vi "Write Datalog.vi"(8 "error in":errorcluster, 9 "Model Name":T1, 10 "Results":T2, 11 "file path (dialog if empty)":path) -> (0 "error in":errorcluster)   [LabVIEW 2017]
uses:
  controls/AC Results.ctl
  controls/Model Name.ctl
  <vilib>/Utility/file.llb/Write Delimited Spreadsheet (string).vi
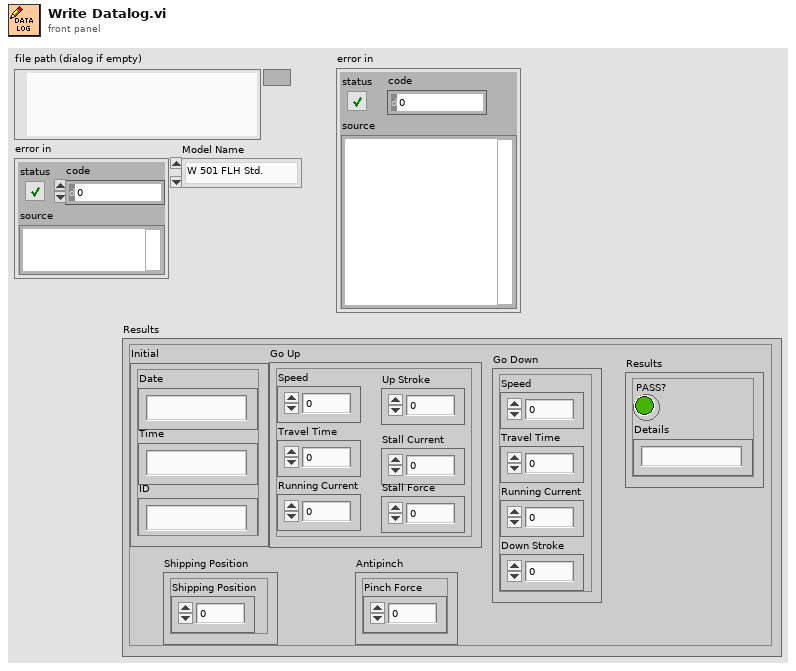
[diagram p1: front panel]
types:
  T1 = typedef "Model Name.ctl" = enum16{"W 501 FLH Std.", "W 501 FRH Std.", "W 601 FR RH Std", "W 601 FR LH Std", "W 601 RR RH Std", "W 601 RR LH Std", "W 601 FR RH AP", "W 601 FR LH AP", "W 601 RR RH AP", "W 601 RR LH AP"}
  T2 = typedef "AC Results.ctl" = cluster{"Initial":cluster{"Date":string, "Time":string, "ID":string}, "Go Up":cluster{"Speed":dbl, "Travel Time":dbl, "Running Current":dbl, "Up Stroke":dbl, "Stall Current":dbl, "Stall Force":dbl}, "Go Down":cluster{"Speed":dbl, "Travel Time":dbl, "Running Current":dbl, "Down Stroke":dbl}, "Shipping Position":cluster{"Shipping Position":dbl}, "Results":cluster{"PASS?":bool, "Details":string}, "Antipinch":cluster{"Pinch Force":dbl}}
  T3 = cluster{"Date":string, "Time":string, "ID":string, string, string, string, string, string, string, string, string, string, string, string, string, string, string, "Details":string}
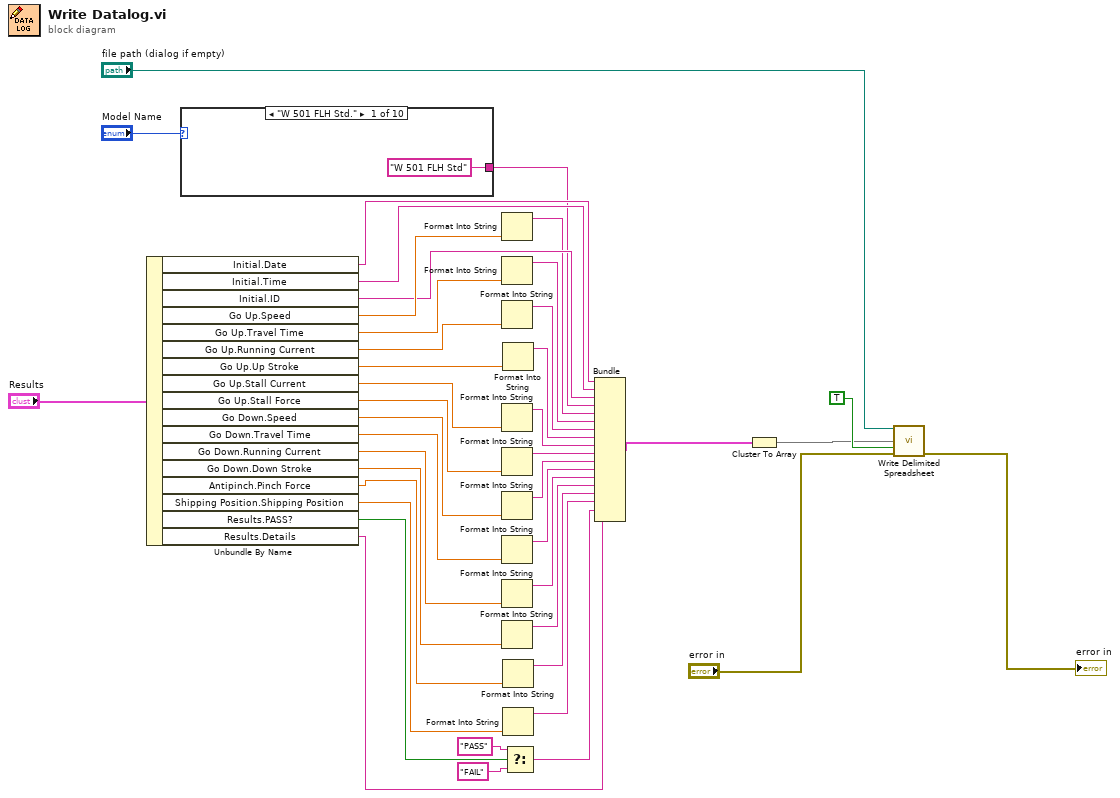
[diagram p0: block diagram]
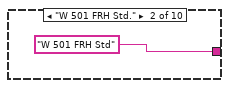
[diagram p2: hidden frame]
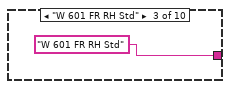
[diagram p3: hidden frame]
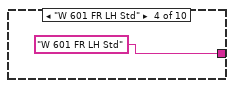
[diagram p4: hidden frame]
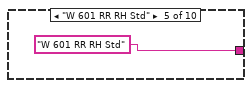
[diagram p5: hidden frame]
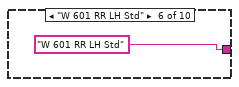
[diagram p6: hidden frame]
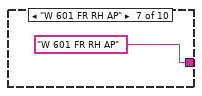
[diagram p7: hidden frame]
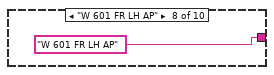
[diagram p8: hidden frame]
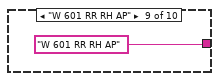
[diagram p9: hidden frame]
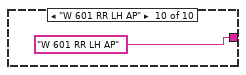
[diagram p10: hidden frame]
diagram:
  n1 = Unbundle By Name("Results") -> ("Initial.Date"=w26:string, "Initial.Time"=w25:string, "Initial.ID"=w24:string, "Go Up.Speed"=w34:dbl, "Go Up.Travel Time"=w33:dbl, "Go Up.Running Current"=w32:dbl, "Go Up.Up Stroke"=w11:dbl, "Go Up.Stall Current"=w31:dbl, "Go Up.Stall Force"=w30:dbl, "Go Down.Speed"=w29:dbl, "Go Down.Travel Time"=w28:dbl, "Go Down.Running Current"=w27:dbl, "Go Down.Down Stroke"=w9:dbl, "Antipinch.Pinch Force"=w4:dbl, "Shipping Position.Shipping Position"=w3:dbl, "Results.PASS?"=w8:bool, "Results.Details"=w7:string)
  n2 = case shown="\"W 501 FLH Std.\"" "Model Name" {
    tunnel: ["W 501 FLH Std" "W 501 FRH Std" "W 601 FR RH Std" "W 601 FR LH Std" "W 601 RR RH Std" "W 601 RR LH Std" "W 601 FR RH AP" "W 601 FR LH AP" "W 601 RR RH AP" "W 601 RR LH AP"] -> w14
    frame "W 501 FLH Std." {
    }
    frame "W 501 FRH Std." {
    }
    frame "W 601 FR RH Std" {
    }
    frame "W 601 FR LH Std" {
    }
    frame "W 601 RR RH Std" {
    }
    frame "W 601 RR LH Std" {
    }
    frame "W 601 FR RH AP" {
    }
    frame "W 601 FR LH AP" {
    }
    frame "W 601 RR RH AP" {
    }
    frame "W 601 RR LH AP" {
    }
  }
  n3 = Format Into String(w34) -> (resulting string=w23:string)  [unwired: 3 in, 1 out]
  n4 = Format Into String(w33) -> (resulting string=w22:string)  [unwired: 3 in, 1 out]
  n5 = Format Into String(w32) -> (resulting string=w21:string)  [unwired: 3 in, 1 out]
  n6 = Format Into String(w31) -> (resulting string=w20:string)  [unwired: 3 in, 1 out]
  n7 = Format Into String(w30) -> (resulting string=w19:string)  [unwired: 3 in, 1 out]
  n8 = Format Into String(w29) -> (resulting string=w18:string)  [unwired: 3 in, 1 out]
  n9 = Format Into String(w28) -> (resulting string=w17:string)  [unwired: 3 in, 1 out]
  n10 = Format Into String(w27) -> (resulting string=w16:string)  [unwired: 3 in, 1 out]
  n11 = Format Into String(w9) -> (resulting string=w5:string)  [unwired: 3 in, 1 out]
  n12 = Format Into String(w11) -> (resulting string=w10:string)  [unwired: 3 in, 1 out]
  n13 = Format Into String(w4) -> (resulting string=w2:string)  [unwired: 3 in, 1 out]
  n14 = Format Into String(w3) -> (resulting string=w1:string)  [unwired: 3 in, 1 out]
  n15 = Select(t="PASS", s=w8, f="FAIL") -> (s? t:f=w6:string)
  n16 = Bundle("Date"=w26, "Time"=w25, "ID"=w24, w14, w23, w22, w21, w10, w20, w19, w18, w17, w16, w5, w2, w1, w6, "Details"=w7) -> (w13:T3)  [unwired: 1 in]
  n17 = Cluster To Array(cluster=w13) -> (array=w12:string[])
  n18 = call-poly <vilib>:"Write Delimited Spreadsheet.vi"("file path (dialog if empty)"="file path (dialog if empty)", "1D data"=w12, "append to file? (new file:F)"=TRUE, "error in (no error)"="error in") -> ("error out"=→"error in":errorcluster)  [unwired: 10 in, 1 out]
